vi "CRYCalc Wave & Value.vi"(8 "Value in":T2={"Name"="", "Curve"=[], "X data"=1, "Y data"=1, "Z data"=1, "X axis"=0, "Y axis"=1, "Z axis"=1, "X unit"="Hz", "Y unit"="", "Z unit"="deg.", "X dB ref"=1.0, "Y dB ref"=1.0, "Z dB ref"=1.0, "single val"=FALSE, "protected"=FALSE, "display X"=TRUE, "display Y"=TRUE, "display Z"=TRUE, "Test Info"="", "Step No."=0, "Plot Settings"={"Color"=0, "Interpolation"=0, "Point Style"=0, "Line Style"=0, "Point Color"=0, "Line Width"=0, "Bar Plot Style"=0, "Fill To"=0}, "AutoProtect"=FALSE} {"Z data" items=["dB", "Lin"]; "X data" items=["dB", "Lin"]; "Y data" items=["dB", "Lin"]; "Z dB ref" format="%.1f"; "Z axis" items=["Log", "Lin"]; "X dB ref" format="%.1f"; "X axis" items=["Log", "Lin"]; "Y axis" items=["Log", "Lin"]; "Y dB ref" format="%.1f"; "Curve"."z" format="%.2f"; "Curve"."y" format="%.2f"; "Curve"."x" format="%.2f"}, 9 "Work in":u16(slide), 10 "Operator":u16(ring) items=["+", "--", "x", "/"], 11 "Wave in":T1={"Waveform"={"X0"=0.0, "dX"=0.0, "Y"=[]}, "X data"=1, "Y data"=1, "Y axis"=1, "X unit"="s", "Y unit"="V", "Y dB ref"=1.0, "display Y"=TRUE, "display X"=TRUE, "Overload?"=FALSE, "Test Info"="", "Step No."=0, "Name"="", "protected"=FALSE, "Sqc history"=[], "Signal Channel ID"=0, "Plot Settings"={"Color"=0, "Interpolation"=0, "Point Style"=0, "Line Style"=0, "Point Color"=0, "Line Width"=0, "Bar Plot Style"=0, "Fill To"=0}, "AutoProtect"=FALSE} {"Y dB ref" format="%.1f"; "Y axis" items=["Log", "Lin"]; "Y data" items=["dB", "Lin"]; "X data" items=["dB", "Lin"]}) -> (3 "Wave out":T1={"Waveform"={"X0"=0.0, "dX"=0.0, "Y"=[]}, "X data"=1, "Y data"=1, "Y axis"=1, "X unit"="s", "Y unit"="V", "Y dB ref"=1.0, "display Y"=TRUE, "display X"=TRUE, "Overload?"=FALSE, "Test Info"="", "Step No."=0, "Name"="", "protected"=FALSE, "Sqc history"=[], "Signal Channel ID"=0, "Plot Settings"={"Color"=0, "Interpolation"=0, "Point Style"=0, "Line Style"=0, "Point Color"=0, "Line Width"=0, "Bar Plot Style"=0, "Fill To"=0}, "AutoProtect"=FALSE} {"Y dB ref" format="%.1f"; "Y axis" items=["Log", "Lin"]; "Y data" items=["dB", "Lin"]; "X data" items=["dB", "Lin"]})   [LabVIEW 2013]
uses:
  Typedef Control/CRYWaveform Cluster.ctl
  Typedef Control/CRYData Cluster.ctl
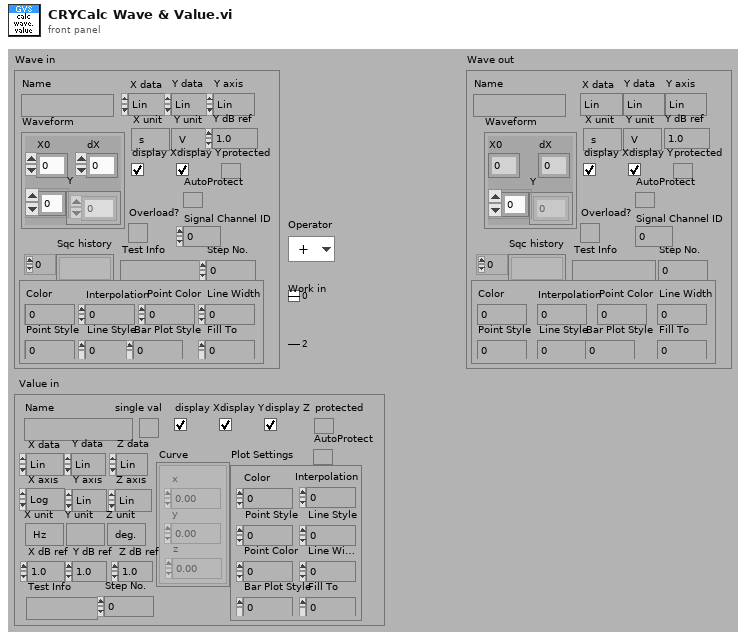
[diagram p1: front panel]
types:
  T1 = typedef "CRYWaveform Cluster.ctl" = cluster{"Waveform":cluster{"X0":dbl, "dX":dbl, "Y":sgl[]}, "X data":u16, "Y data":u16, "Y axis":u16, "X unit":string, "Y unit":string, "Y dB ref":dbl, "display Y":bool, "display X":bool, "Overload?":bool, "Test Info":string, "Step No.":i32, "Name":string, "protected":bool, "Sqc history":string[], "Signal Channel ID":i32, "Plot Settings":cluster{"Color":u32, "Interpolation":u8, "Point Style":u8, "Line Style":u8, "Point Color":u32, "Line Width":u8, "Bar Plot Style":u8, "Fill To":i16}, "AutoProtect":bool}
  T2 = typedef "CRYData Cluster.ctl" = cluster{"Name":string, "Curve":cluster{"x":dbl, "y":dbl, "z":dbl}[], "X data":u16, "Y data":u16, "Z data":u16, "X axis":u16, "Y axis":u16, "Z axis":u16, "X unit":string, "Y unit":string, "Z unit":string, "X dB ref":dbl, "Y dB ref":dbl, "Z dB ref":dbl, "single val":bool, "protected":bool, "display X":bool, "display Y":bool, "display Z":bool, "Test Info":string, "Step No.":i32, "Plot Settings":cluster{"Color":u32, "Interpolation":u8, "Point Style":u8, "Line Style":u8, "Point Color":u32, "Line Width":u8, "Bar Plot Style":u8, "Fill To":i16}, "AutoProtect":bool}
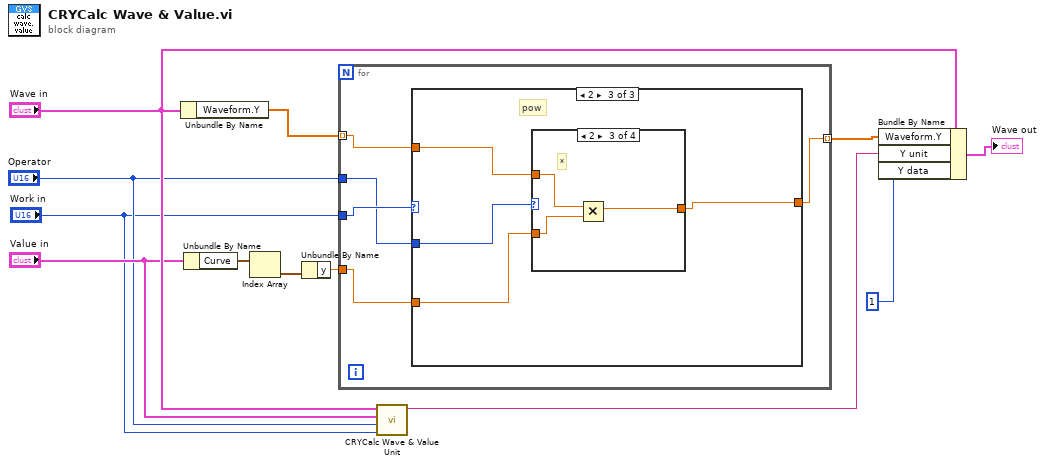
[diagram p0: block diagram]
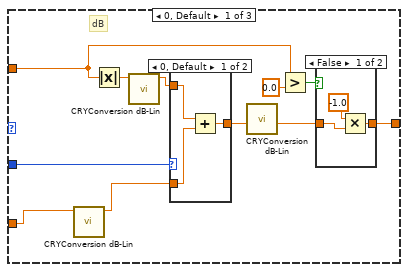
[diagram p2: hidden frame]
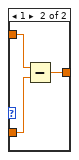
[diagram p4: hidden frame]
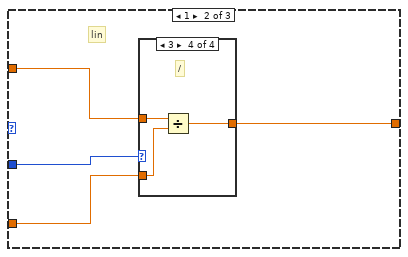
[diagram p5: hidden frame]
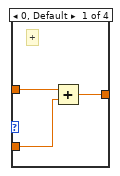
[diagram p6: hidden frame]
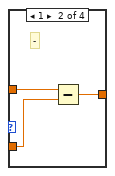
[diagram p7: hidden frame]
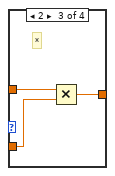
[diagram p8: hidden frame]
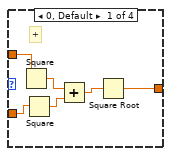
[diagram p9: hidden frame]
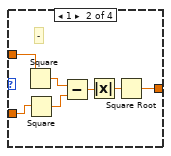
[diagram p10: hidden frame]
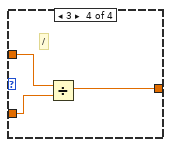
[diagram p11: hidden frame]
diagram:
  n1 = Unbundle By Name("Wave in") -> ("Waveform.Y"=w10:sgl[])
  n2 = Unbundle By Name("Value in") -> ("Curve"=w12:cluster{"x":dbl, "y":dbl, "z":dbl}[])
  n3 = Index Array(array=w12) -> (element=w11:cluster{"x":dbl, "y":dbl, "z":dbl})  [unwired: 1 in]
  n4 = Unbundle By Name(w11) -> ("y"=w9:dbl)
  n5 = for {
    tunnel: "Operator" -> [w15]
    tunnel: w10 -> [w17] mode=indexing
    tunnel: w9 -> [w13]
    tunnel: "Work in" -> [w16]
    tunnel: [w14] -> w1 mode=indexing
    n6 = case shown="2" w16 {
      tunnel: w15 -> [w28 w42 w58]
      tunnel: w13 -> [w19 w40 w57]
      tunnel: w17 -> [w24 w41 w56]
      tunnel: [w21 w39 w55] -> w14
      frame 0, Default {
        # "dB"
        n7 = call "CRYConversion dB-Lin.vi"("Lin In"=w19) -> ("Log Out"=w18:dbl)  [unwired: 5 in, 3 out]
        n8 = Absolute Value(x=w24) -> (abs(x)=w25:sgl)
        n9 = call "CRYConversion dB-Lin.vi"("Lin In"=w25) -> ("Log Out"=w26:dbl)  [unwired: 5 in, 3 out]
        n10 = case shown="0, Default" w28 {
          tunnel: w18 -> [w34 w36]
          tunnel: w26 -> [w35 w37]
          tunnel: [w33 w38] -> w27
          frame 0, Default {
            n11 = Add(x=w35, y=w34) -> (x+y=w33:dbl)
          }
          frame 1 {
            n12 = Subtract(x=w37, y=w36) -> (x-y=w38:dbl)
          }
        }
        n13 = call "CRYConversion dB-Lin.vi"("Log In"=w27) -> ("Lin Out"=w20:dbl)  [unwired: 5 in, 3 out]
        n14 = Greater?(x=w24, y=sgl 0.0) -> (0:w22:bool)
        n15 = case shown="False" w22 {
          tunnel: [w31 w32] -> w21
          tunnel: w20 -> [w30 w32]
          frame False {
            n16 = Multiply(x=-1.0, y=w30) -> (x*y=w31:dbl)
          }
          frame True {
          }
        }
      }
      frame 1 {
        # "lin"
        n17 = case shown="3" w42 {
          tunnel: w41 -> [w45 w48 w51 w53]
          tunnel: w40 -> [w44 w47 w50 w52]
          tunnel: [w43 w46 w49 w54] -> w39
          frame 0, Default {
            # "+"
            n18 = Add(x=w45, y=w44) -> (x+y=w43:dbl)
          }
          frame 1 {
            # "-"
            n19 = Subtract(x=w48, y=w47) -> (x-y=w46:dbl)
          }
          frame 2 {
            # "*"
            n20 = Multiply(x=w51, y=w50) -> (x*y=w49:dbl)
          }
          frame 3 {
            # "/"
            n21 = Divide(x=w53, y=w52) -> (x/y=w54:dbl)
          }
        }
      }
      frame 2 {
        # "pow"
        n22 = case shown="2" w58 {
          tunnel: w56 -> [w64 w71 w73 w76]
          tunnel: w57 -> [w63 w70 w74 w77]
          tunnel: [w59 w65 w72 w75] -> w55
          frame 0, Default {
            # "+"
            n23 = Square(x=w64) -> (x^2=w62:sgl)
            n24 = Square(x=w63) -> (x^2=w61:dbl)
            n25 = Add(x=w62, y=w61) -> (x+y=w60:dbl)
            n26 = Square Root(x=w60) -> (sqrt(x)=w59:dbl)
          }
          frame 1 {
            # "-"
            n27 = Square(x=w71) -> (x^2=w69:sgl)
            n28 = Square(x=w70) -> (x^2=w68:dbl)
            n29 = Subtract(x=w69, y=w68) -> (x-y=w67:dbl)
            n30 = Absolute Value(x=w67) -> (abs(x)=w66:dbl)
            n31 = Square Root(x=w66) -> (sqrt(x)=w65:dbl)
          }
          frame 2 {
            # "*"
            n32 = Multiply(x=w73, y=w74) -> (x*y=w72:dbl)
          }
          frame 3 {
            # "/"
            n33 = Divide(x=w76, y=w77) -> (x/y=w75:dbl)
          }
        }
      }
    }
  }
  n34 = call "CRYCalc Wave & Value Unit.vi"("Work in"="Work in", "Operator"="Operator", "Value in"="Value in", "Wave in"="Wave in") -> ("Y unit"=w2:string)  [unwired: 4 in, 3 out]
  n35 = Bundle By Name(cluster="Wave in", "Waveform.Y"=w1, "Y unit"=w2, "Y data"=u16 1) -> (→"Wave out":T1)
